vi "steps to um.vi"(7 "axis (default: fine)":enum16{"fine", "coarse"}(ring), 8 "steps":dbl) -> (2 "position (microns)":dbl[unit])   [LabVIEW 2009]
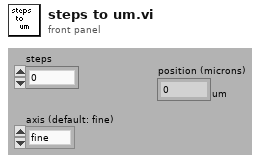
[diagram p1: front panel]
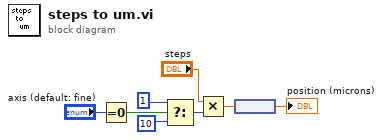
[diagram p0: block diagram]
diagram:
  n1 = Equal To 0?(x="axis (default: fine)") -> (x = 0?=w7:bool)
  n2 = Select(t=i8 1, s=w7, f=i8 10 ("y")) -> (s? t:f=w4:i8)
  n3 = Multiply(x="steps", y=w4) -> (x*y=w2:dbl)
  n4 = node(w2) -> (→"position (microns)":dbl[unit])
